vi "ad start scan v.vi"(0 "adh":i32, 1 "chav":i32, 2 "rangev":i32, 5 "sample_rate":dbl, 7 "posthist":u32, 9 "chac":u32, 11 "error in (no error)":errorcluster, 12 "rangec":u32) -> (3 "chav out":i32, 4 "rangev out":i32, 6 "function return":i32, 15 "error out":errorcluster)   [LabVIEW 2021, in "libad4.lvlib"]
doc: "ad_start_scan_v (int32_t adh, double sample_rate, uint32_t posthist,\n uint32_t chac, int32_t *chav,\n uint32_t rangec, int32_t *rangev);"
uses:
  <userlib>/libad4/libad4.lvlib
  <userlib>/libad4/libad4.dll
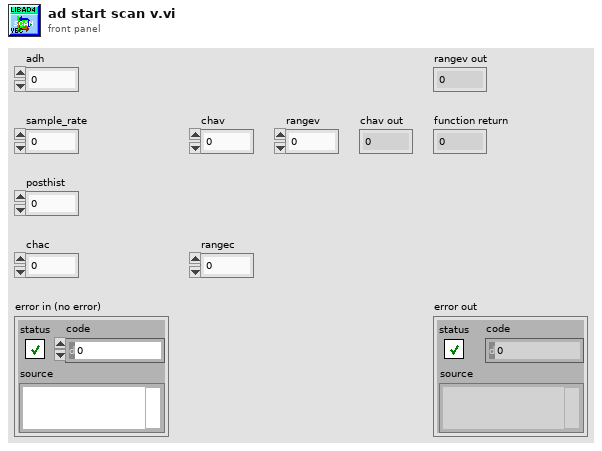
[diagram p1: front panel]
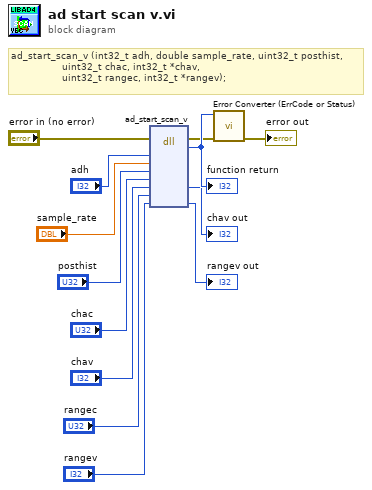
[diagram p0: block diagram]
diagram:
  # "ad_start_scan_v (int32_t adh, double sample_rate, uint32_t posthist,\n                 uint32_t chac, int32_t *chav,\n                 uint32_t rangec, int32_t *rangev);"
  n1 = dll-call lib="C:/Program Files/National Instruments/LabVIEW 2021/user.lib/libad4/libad4.*" fn="ad_start_scan_v"(error in="error in (no error)", "adh"="adh", "sample_rate"="sample_rate", "posthist"="posthist", "chac"="chac", "chav"="chav", "rangec"="rangec", "rangev"="rangev") -> (error out=w2:errorcluster, w13:i32, "chav"=→"chav out":i32, "rangev"=→"rangev out":i32)  [unwired: 7 in, 1 out]
  "function return" <- w13
  n2 = call <userlib>:"Error Converter (ErrCode or Status).vi"("error in (no error)"=w2, "error code"=w13) -> ("error out"=→"error out":errorcluster)  [unwired: 9 in]
